vi "文本转ascii.vi"(11 "文本输入":string) -> (2 "字符串":string, 3 "报错输出":bool)   [LabVIEW 2012]
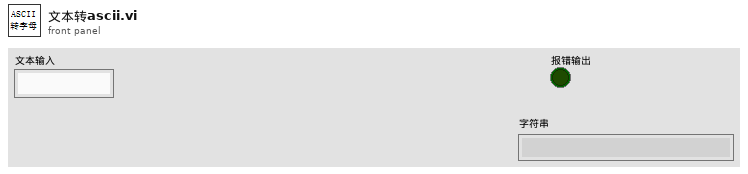
[diagram p1: front panel]
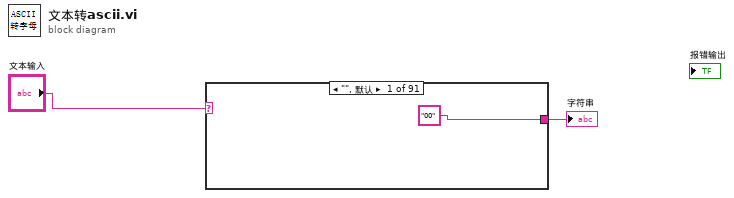
[diagram p0: block diagram]
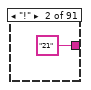
[diagram p2: hidden frame]
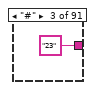
[diagram p3: hidden frame]
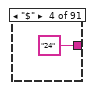
[diagram p4: hidden frame]
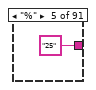
[diagram p5: hidden frame]
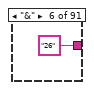
[diagram p6: hidden frame]
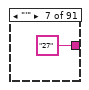
[diagram p7: hidden frame]
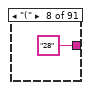
[diagram p8: hidden frame]
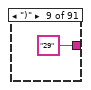
[diagram p9: hidden frame]
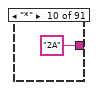
[diagram p10: hidden frame]
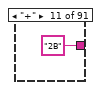
[diagram p11: hidden frame]
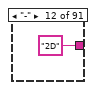
[diagram p12: hidden frame]
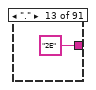
[diagram p13: hidden frame]
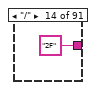
[diagram p14: hidden frame]
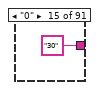
[diagram p15: hidden frame]
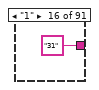
[diagram p16: hidden frame]
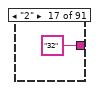
[diagram p17: hidden frame]
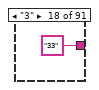
[diagram p18: hidden frame]
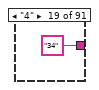
[diagram p19: hidden frame]
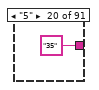
[diagram p20: hidden frame]
diagram:
  n1 = case shown="\"\", 默认" "文本输入" {
    tunnel: ["00" "21" "23" "24" "25" "26" "27" "28" "29" "2A" "2B" "2D" "2E" "2F" "30" "31" "32" "33" "34" "35" "36" "37" "38" "39" "3A" "3B" "3C" "3D" "3E" "3F" "40" "41" "42" "43" "44" "45" "46" "47" "48" "49" "4A" "4B" "4C" "4D" "4E" "4F" "50" "51" "52" "53" "54" "55" "56" "57" "58" "59" "5A" "5B" "5D" "5E" "5F" "60" "61" "62" "63" "64" "65" "66" "67" "68" "69" "6A" "6B" "6C" "6D" "6E" "6F" "70" "71" "72" "73" "74" "75" "76" "77" "78" "79" "7A" "7B" "7C" "7D"] -> w2
    frame "", Default {
    }
    frame "!" {
    }
    frame "#" {
    }
    frame "$" {
    }
    frame "%" {
    }
    frame "&" {
    }
    frame "'" {
    }
    frame "(" {
    }
    frame ")" {
    }
    frame "*" {
    }
    frame "+" {
    }
    frame "-" {
    }
    frame "." {
    }
    frame "/" {
    }
    frame "0" {
    }
    frame "1" {
    }
    frame "2" {
    }
    frame "3" {
    }
    frame "4" {
    }
    frame "5" {
    }
    frame "6" {
    }
    frame "7" {
    }
    frame "8" {
    }
    frame "9" {
    }
    frame ":" {
    }
    frame ";" {
    }
    frame "<" {
    }
    frame "=" {
    }
    frame ">" {
    }
    frame "?" {
    }
    frame "@" {
    }
    frame "A" {
    }
    frame "B" {
    }
    frame "C" {
    }
    frame "D" {
    }
    frame "E" {
    }
    frame "F" {
    }
    frame "G" {
    }
    frame "H" {
    }
    frame "I" {
    }
    frame "J" {
    }
    frame "K" {
    }
    frame "L" {
    }
    frame "M" {
    }
    frame "N" {
    }
    frame "O" {
    }
    frame "P" {
    }
    frame "Q" {
    }
    frame "R" {
    }
    frame "S" {
    }
    frame "T" {
    }
    frame "U" {
    }
    frame "V" {
    }
    frame "W" {
    }
    frame "X" {
    }
    frame "Y" {
    }
    frame "Z" {
    }
    frame "[" {
    }
    frame "]" {
    }
    frame "^" {
    }
    frame "_" {
    }
    frame "`" {
    }
    frame "a" {
    }
    frame "b" {
    }
    frame "c" {
    }
    frame "d" {
    }
    frame "e" {
    }
    frame "f" {
    }
    frame "g" {
    }
    frame "h" {
    }
    frame "i" {
    }
    frame "j" {
    }
    frame "k" {
    }
    frame "l" {
    }
    frame "m" {
    }
    frame "n" {
    }
    frame "o" {
    }
    frame "p" {
    }
    frame "q" {
    }
    frame "r" {
    }
    frame "s" {
    }
    frame "t" {
    }
    frame "u" {
    }
    frame "v" {
    }
    frame "w" {
    }
    frame "x" {
    }
    frame "y" {
    }
    frame "z" {
    }
    frame "{" {
    }
    frame "|" {
    }
    frame "}" {
    }
  }
  "字符串" <- w2
